vi "Drive_Hardware_Begin.vi"() -> ()   [LabVIEW 2019]
uses:
  <vilib>/Rock Robotics/WPI/ThirdParty/Phoenix-LabVIEW/Motor Controller/Controls/CTRE_Phoenix_MotorControl_BaseConfigurables.ctl
  <vilib>/Rock Robotics/WPI/ThirdParty/Phoenix-LabVIEW/Motor Controller/Controls/CTRE_Phoenix_MotorControl_VelocityMeasurementPeriod.ctl
  <vilib>/Rock Robotics/WPI/ThirdParty/Phoenix-LabVIEW/Motor Controller/Controls/CTRE_Phoenix_MotorControl_SlotStructure.ctl
  <vilib>/Rock Robotics/WPI/ThirdParty/Phoenix-LabVIEW/Motor Controller/Controls/CTRE_Phoenix_MotorControl_FilterStruct.ctl
  <vilib>/Rock Robotics/WPI/ThirdParty/Phoenix-LabVIEW/Motor Controller/Controls/CTRE_Phoenix_MotorControl_RemoteSourceType.ctl
  <vilib>/Rock Robotics/WPI/ThirdParty/Phoenix-LabVIEW/Controls/CTRE_Phoenix_CustomParamConfiguration.ctl
  <vilib>/Rock Robotics/WPI/ThirdParty/Phoenix-LabVIEW/Motor Controller/Controls/CTRE_Phoenix_MotorControl_FeedbackDevice_TalonFX.ctl
  <vilib>/Rock Robotics/WPI/ThirdParty/Phoenix-LabVIEW/Motor Controller/Controls/CTRE_Phoenix_MotorControl_LimitSwitchNormal.ctl
  <vilib>/Rock Robotics/WPI/ThirdParty/Phoenix-LabVIEW/Motor Controller/Controls/CTRE_Phoenix_MotorControl_LimitSwitchSource_Local.ctl
  <vilib>/Rock Robotics/WPI/ThirdParty/Phoenix-LabVIEW/Motor Controller/Controls/CTRE_Phoenix_MotorControl_SupplyCurrentLimitConfiguration.ctl
  <vilib>/Rock Robotics/WPI/ThirdParty/Phoenix-LabVIEW/Motor Controller/Controls/CTRE_Phoenix_MotorControl_StatorCurrentLimitConfiguration.ctl
  <vilib>/Rock Robotics/WPI/ThirdParty/Phoenix-LabVIEW/Motor Controller/Controls/CTRE_Phoenix_MotorControl_MotorCommutation_TalonFX.ctl
  <vilib>/Rock Robotics/WPI/ThirdParty/Phoenix-LabVIEW/CANCoder/Controls/CTRE_Phoenix_CANcoder_AbsoluteSensorRange.ctl
  <vilib>/Rock Robotics/WPI/ThirdParty/Phoenix-LabVIEW/CANCoder/Controls/CTRE_Phoenix_CANcoder_SensorInitializationStrategy.ctl
  <vilib>/Rock Robotics/WPI/ThirdParty/Phoenix-LabVIEW/Motor Controller/Controls/CTRE_Phoenix_MotorControl_TalonFXInvertType.ctl
  <vilib>/Rock Robotics/WPI/ThirdParty/Phoenix-LabVIEW/Motor Controller/Controls/CTRE_Phoenix_MotorControl_NeutralMode.ctl
  <vilib>/Rock Robotics/WPI/ThirdParty/Phoenix-LabVIEW/Pigeon IMU/CTRE_PigeonIMU_Open_TalonSRX.vi
  Globals/Drive_Globals.vi
panel:
  in  "Talon FX Configurables":T15={"Base Configurables"={"openLoopRamp"=0.0, "closedLoopRamp"=0.0, "peakOutputForward"=1.0, "peakOutputReverse"=-1.0, "nominalOutputForward"=0.0, "nominalOutputReverse"=0.0, "neutralDeadband"=0.0, "voltageCompSaturation"=0.0, "voltageMeasurementFilter"=32, "velocityMeasurementPeriod"=100, "velocityMeasurementWindow"=64, "forwardSoftLimitThreshold"=0, "reverseSoftLimitThreshold"=0, "forwardSoftLimitEnable"=FALSE, "reverseSoftLimitEnable"=FALSE, "slot0"={"P"=0.0, "I"=0.0, "D"=0.0, "F"=0.0, "integralZone"=0.0, "allowableClosedLoopError"=0, "maxIntegralAccumulator"=0.0, "closedLoopPeakOutput"=1.0, "closedLoopPeriod"=1}, "slot1"={"P"=0.0, "I"=0.0, "D"=0.0, "F"=0.0, "integralZone"=0.0, "allowableClosedLoopError"=0, "maxIntegralAccumulator"=0.0, "closedLoopPeakOutput"=1.0, "closedLoopPeriod"=1}, "slot2"={"P"=0.0, "I"=0.0, "D"=0.0, "F"=0.0, "integralZone"=0.0, "allowableClosedLoopError"=0, "maxIntegralAccumulator"=0.0, "closedLoopPeakOutput"=1.0, "closedLoopPeriod"=1}, "slot3"={"P"=0.0, "I"=0.0, "D"=0.0, "F"=0.0, "integralZone"=0.0, "allowableClosedLoopError"=0, "maxIntegralAccumulator"=0.0, "closedLoopPeakOutput"=1.0, "closedLoopPeriod"=1}, "auxPIDPolarity"=FALSE, "remoteFilter0"={"remoteSensorDeviceID"=0, "remoteSensorSource"=enum."Off"}, "remoteFilter1"={"remoteSensorDeviceID"=0, "remoteSensorSource"=enum."Off"}, "motionCruiseVelocity"=0, "motionAcceleration"=0, "motionProfileTrajectoryPeriod"=0, "feedbackNotContinuous"=FALSE, "remoteSensorClosedLoopDisableNeutralOnLOS"=FALSE, "clearPositionOnLimitF"=FALSE, "clearPositionOnLimitR"=FALSE, "clearPositionOnQuadIdx"=FALSE, "limitSwitchDisableNeutralOnLOS"=FALSE, "softLimitDisableNeutralOnLOS"=FALSE, "pulseWidthPeriod_EdgesPerRot"=1, "pulseWidthPeriod_FilterWindowSz"=1, "customParam"={"customParam0"=0, "customParam1"=0}, "trajectoryInterpolationEnable"=TRUE}, "primaryPID"={"selectedFeedbackCoefficient"=1.0, "selectedFeedbackSensor"=1}, "auxiliaryPID"={"selectedFeedbackCoefficient"=1.0, "selectedFeedbackSensor"=1}, "forwardLimitSwitchNormal"=enum."Normally Open", "reverseLimitSwitchNormal"=enum."Normally Open", "forwardLimitSwitchDeviceID"=0, "reverseLimitSwitchDeviceID"=0, "forwardLimitSwitchSource"=enum."Feedback Connector", "reverseLimitSwitchSource"=enum."Feedback Connector", "sum0Term"=1, "sum1Term"=1, "diff0Term"=1, "diff1Term"=1, "Supply Current Limit Configuration"={"Enable?"=FALSE, "Current Limit"=0.0, "Threshold Current"=0.0, "Threshold Time"=0.0}, "Stator Current Limit Configuration"={"Enable?"=FALSE, "Current Limit"=0.0, "Threshold Current"=0.0, "Threshold Time"=0.0}, "Motor Commutation"=enum."Trapezoidal", "Absolute Sensor Range"=enum."Unsigned [0 to 360)", "Integrated Sensor Offset (Degrees)"=0.0, "Sensor Initialization Strategy"=enum."Boot To Zero"} {"Base Configurables"."velocityMeasurementPeriod" items=["Period_1ms"=1, "Period_2ms"=2, "Period_5ms"=5, "Period_10ms"=10, "Period_20ms"=20, "Period_25ms"=25, "Period_50ms"=50, "Period_100ms"=100]; "primaryPID"."selectedFeedbackSensor" items=["Integrated Sensor"=1, "Sensor Sum (S0 + S1)"=9, "Sensor Difference (D0 - D1)"=10, "Remote Source 0"=11, "Remote Source 1"=12, "None"=14, "Software Emulated"=15]; "auxiliaryPID"."selectedFeedbackSensor" items=["Integrated Sensor"=1, "Sensor Sum (S0 + S1)"=9, "Sensor Difference (D0 - D1)"=10, "Remote Source 0"=11, "Remote Source 1"=12, "None"=14, "Software Emulated"=15]; "sum0Term" items=["Integrated Sensor"=1, "Sensor Sum (S0 + S1)"=9, "Sensor Difference (D0 - D1)"=10, "Remote Source 0"=11, "Remote Source 1"=12, "None"=14, "Software Emulated"=15]; "sum1Term" items=["Integrated Sensor"=1, "Sensor Sum (S0 + S1)"=9, "Sensor Difference (D0 - D1)"=10, "Remote Source 0"=11, "Remote Source 1"=12, "None"=14, "Software Emulated"=15]; "diff0Term" items=["Integrated Sensor"=1, "Sensor Sum (S0 + S1)"=9, "Sensor Difference (D0 - D1)"=10, "Remote Source 0"=11, "Remote Source 1"=12, "None"=14, "Software Emulated"=15]; "diff1Term" items=["Integrated Sensor"=1, "Sensor Sum (S0 + S1)"=9, "Sensor Difference (D0 - D1)"=10, "Remote Source 0"=11, "Remote Source 1"=12, "None"=14, "Software Emulated"=15]}
  # "False: Primary Output = PID[0] + PID[1]  ---  Auxiliary Output = PID[0] - PID[1]\nTrue:  Primary Output = PID[0] - PID[1] --- Auxiliary Output = PID[0] + PID[1]"
  # "Enable the motion profile executor to perform linear interpolation between profile points.  Defaults to True."
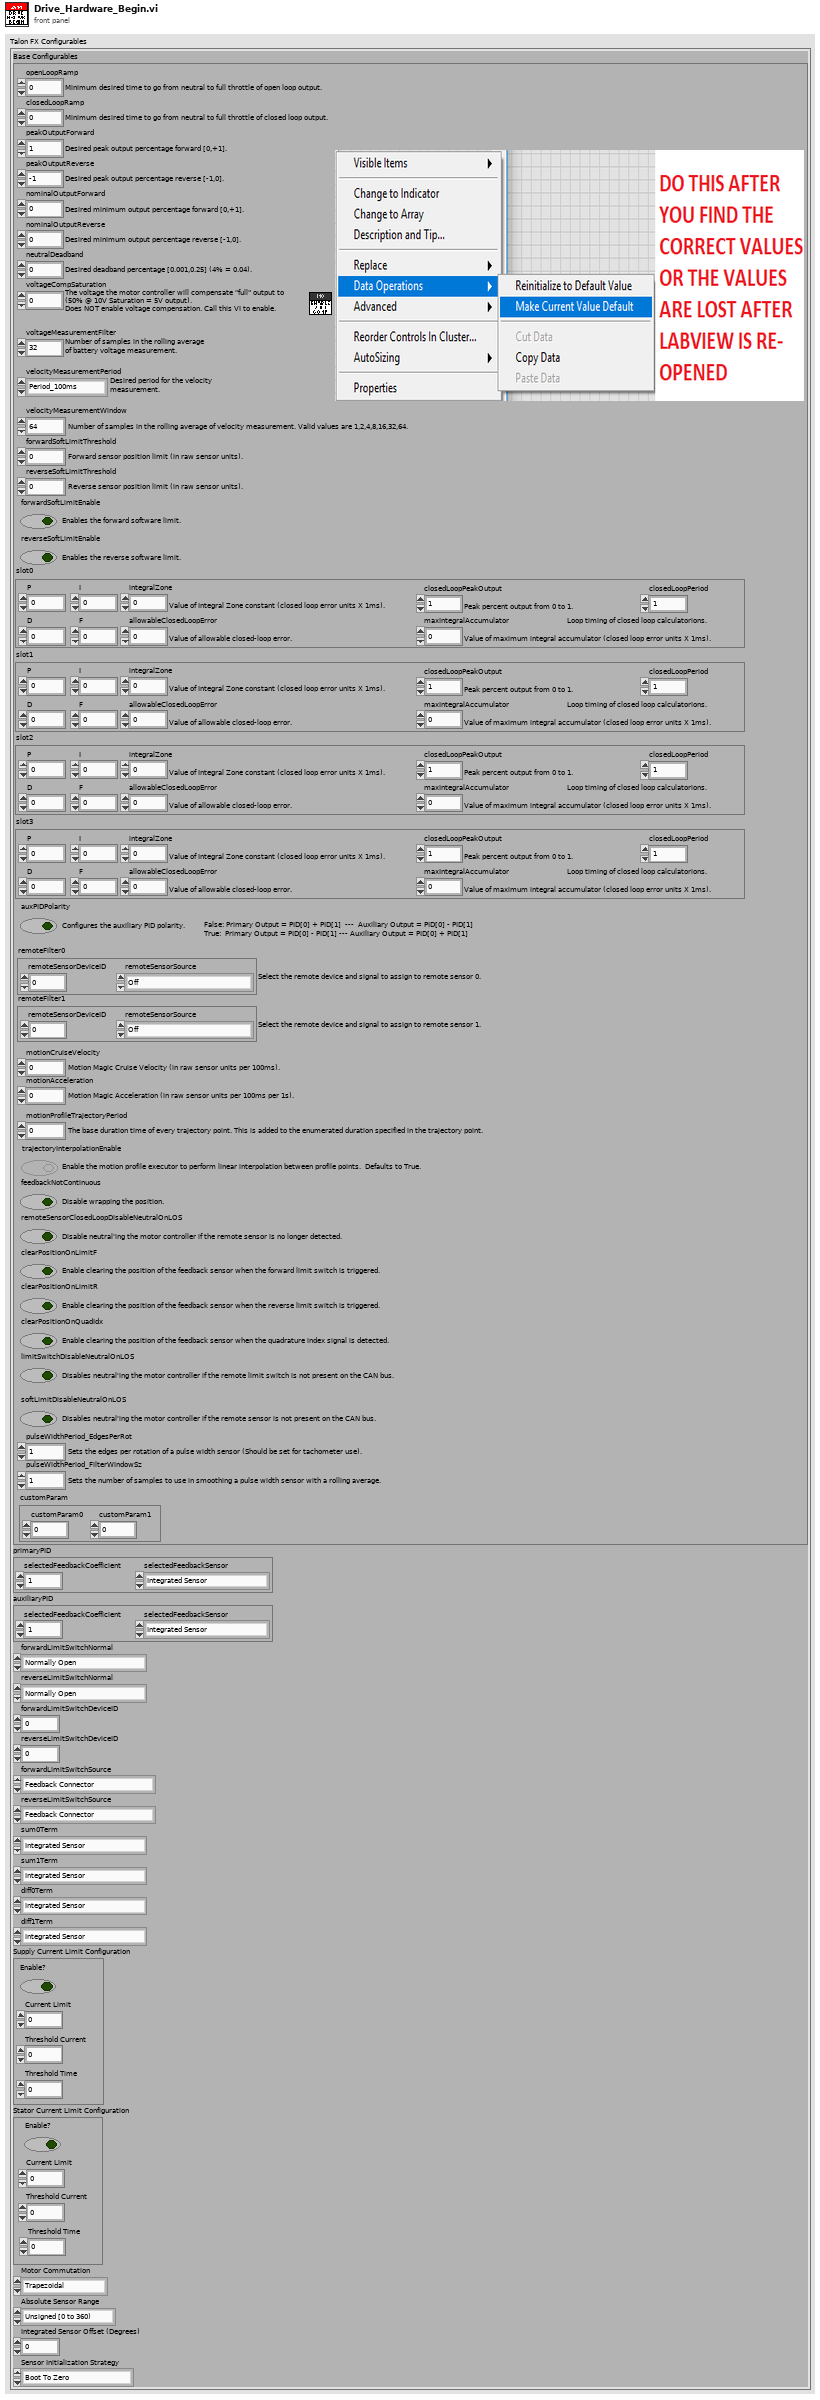
[diagram p1: front panel]
types:
  T1 = typedef "CTRE_Phoenix_MotorControl_BaseConfigurables.ctl" = cluster{"openLoopRamp":dbl, "closedLoopRamp":dbl, "peakOutputForward":dbl, "peakOutputReverse":dbl, "nominalOutputForward":dbl, "nominalOutputReverse":dbl, "neutralDeadband":dbl, "voltageCompSaturation":dbl, "voltageMeasurementFilter":i32, "velocityMeasurementPeriod":T2, "velocityMeasurementWindow":i32, "forwardSoftLimitThreshold":i32, "reverseSoftLimitThreshold":i32, "forwardSoftLimitEnable":bool, "reverseSoftLimitEnable":bool, "slot0":T3, "slot1":T3, "slot2":T3, "slot3":T3, "auxPIDPolarity":bool, "remoteFilter0":T4, "remoteFilter1":T4, "motionCruiseVelocity":i32, "motionAcceleration":i32, "motionProfileTrajectoryPeriod":i32, "feedbackNotContinuous":bool, "remoteSensorClosedLoopDisableNeutralOnLOS":bool, "clearPositionOnLimitF":bool, "clearPositionOnLimitR":bool, "clearPositionOnQuadIdx":bool, "limitSwitchDisableNeutralOnLOS":bool, "softLimitDisableNeutralOnLOS":bool, "pulseWidthPeriod_EdgesPerRot":i32, "pulseWidthPeriod_FilterWindowSz":i32, "customParam":T6, "trajectoryInterpolationEnable":bool}
  T2 = typedef "CTRE_Phoenix_MotorControl_VelocityMeasurementPeriod.ctl" = u16
  T3 = typedef "CTRE_Phoenix_MotorControl_SlotStructure.ctl" = cluster{"P":dbl, "I":dbl, "D":dbl, "F":dbl, "integralZone":dbl, "allowableClosedLoopError":i32, "maxIntegralAccumulator":dbl, "closedLoopPeakOutput":dbl, "closedLoopPeriod":i32}
  T4 = typedef "CTRE_Phoenix_MotorControl_FilterStruct.ctl" = cluster{"remoteSensorDeviceID":u8, "remoteSensorSource":T5}
  T5 = typedef "CTRE_Phoenix_MotorControl_RemoteSourceType.ctl" = enum16{"Off", "Talon SRX Selected Sensor", "Pigeon IMU Yaw", "Pigeon IMU Pitch", "Pigeon IMU Roll", "CANifier Quadrature", "CANifier PWM Input 0", "CANifier PWM Input 1", "CANifier PWM Input 2", "CANifier PWM Input 3", "Gadgeteer Pigeon Yaw", "Gadgeteer Pigeon Pitch", "Gadgeteer Pigeon Roll", "CANCoder"}
  T6 = typedef "CTRE_Phoenix_CustomParamConfiguration.ctl" = cluster{"customParam0":i32, "customParam1":i32}
  T7 = typedef "CTRE_Phoenix_MotorControl_FeedbackDevice_TalonFX.ctl" = i8
  T8 = typedef "CTRE_Phoenix_MotorControl_LimitSwitchNormal.ctl" = enum16{"Normally Open", "Normally Closed", "Disabled"}
  T9 = typedef "CTRE_Phoenix_MotorControl_LimitSwitchSource_Local.ctl" = enum16{"Feedback Connector", "Remote Talon SRX", "Remote CANifier", "Deactivated"}
  T10 = typedef "CTRE_Phoenix_MotorControl_SupplyCurrentLimitConfiguration.ctl" = cluster{"Enable?":bool, "Current Limit":dbl, "Threshold Current":dbl, "Threshold Time":dbl}
  T11 = typedef "CTRE_Phoenix_MotorControl_StatorCurrentLimitConfiguration.ctl" = cluster{"Enable?":bool, "Current Limit":dbl, "Threshold Current":dbl, "Threshold Time":dbl}
  T12 = typedef "CTRE_Phoenix_MotorControl_MotorCommutation_TalonFX.ctl" = enum16{"Trapezoidal"}
  T13 = typedef "CTRE_Phoenix_CANcoder_AbsoluteSensorRange.ctl" = enum16{"Unsigned [0 to 360)", "Signed [-180 to +180)"}
  T14 = typedef "CTRE_Phoenix_CANcoder_SensorInitializationStrategy.ctl" = enum16{"Boot To Zero", "Boot To Absolute Position"}
  T15 = cluster{"Base Configurables":T1, "primaryPID":cluster{"selectedFeedbackCoefficient":dbl, "selectedFeedbackSensor":T7}, "auxiliaryPID":cluster{"selectedFeedbackCoefficient":dbl, "selectedFeedbackSensor":T7}, "forwardLimitSwitchNormal":T8, "reverseLimitSwitchNormal":T8, "forwardLimitSwitchDeviceID":i32, "reverseLimitSwitchDeviceID":i32, "forwardLimitSwitchSource":T9, "reverseLimitSwitchSource":T9, "sum0Term":T7, "sum1Term":T7, "diff0Term":T7, "diff1Term":T7, "Supply Current Limit Configuration":T10, "Stator Current Limit Configuration":T11, "Motor Commutation":T12, "Absolute Sensor Range":T13, "Integrated Sensor Offset (Degrees)":dbl, "Sensor Initialization Strategy":T14}
  T16 = typedef "CTRE_Phoenix_MotorControl_TalonFXInvertType.ctl" = enum16{"Counter-Clockwise", "Clockwise"}
  T17 = typedef "CTRE_Phoenix_MotorControl_NeutralMode.ctl" = enum8{"EEPROMSetting", "Override to Coast", "Override to Brake"}
  T18 = typedef "WPI_MotorControlDeviceRef.ctl" = cluster{"DeviceStatus":errorcluster, "Type":T19, "PWM":cluster{"PWM Channel":T20, "DeadBand":T21}, "CAN":cluster{"Device Number":u8, "SetOutput VI Ref":variant, "GetOutput VI Ref":variant, "Enable VI Ref":variant, "Disable VI Ref":variant, "Data":variant}, "Invert":bool, "DIO PWM":cluster{"PWM \"Enable\" Channel":T20, "DIOChannel":T22, "PWM Rate":dbl}}
  T19 = typedef "WPI_MotorControlType.ctl" = enum16{"PWM", "CAN", "DIO PWM"}
  T20 = typedef "FPGA_DIOPWMChannel.ctl" = enum8{"PWM 0", "PWM 1", "PWM 2", "PWM 3", "PWM 4", "PWM 5", "PWM 6", "PWM 7", "PWM 8", "PWM 9", "PWM MXP 0", "PWM MXP 1", "PWM MXP 2", "PWM MXP 3", "PWM MXP 4", "PWM MXP 5", "PWM MXP 6", "PWM MXP 7", "PWM MXP 8", "PWM MXP 9", "Invalid"}
  T21 = typedef "WPI_PWMDeadband.ctl" = cluster{"Name":string, "maxPositivePwm":i32, "minPositivePwm":i32, "centerPwm":i32, "maxNegativePwm":i32, "minNegativePwm":i32, "angularRange":u16}
  T22 = typedef "FPGA_DIOChannel.ctl" = enum8{"DIO 0", "DIO 1", "DIO 2", "DIO 3", "DIO 4", "DIO 5", "DIO 6", "DIO 7", "DIO 8", "DIO 9", "DIO MXP 0", "DIO MXP 1", "DIO MXP 2", "DIO MXP 3", "DIO MXP 4", "DIO MXP 5", "DIO MXP 6", "DIO MXP 7", "DIO MXP 8", "DIO MXP 9", "DIO MXP 10", "DIO MXP 11", "DIO MXP 12", "DIO MXP 13", "DIO MXP 14", "DIO MXP 15", "SPI Port CS1", "SPI Port CS2", "SPI Port CS3", "SPI Port MISO", "SPI Port MOSI", "Invalid"}
  T23 = typedef "CTRE_PigeonIMU_DeviceRef.ctl" = cluster{"DeviceStatus":errorcluster, "Device Number":u8, "Type":T24, "Device ID":u32, "Handle":u64, "UsageFrame":u32, "Library Path":path}
  T24 = typedef "CTRE_PigeonIMU_ConnectionType.ctl" = u32
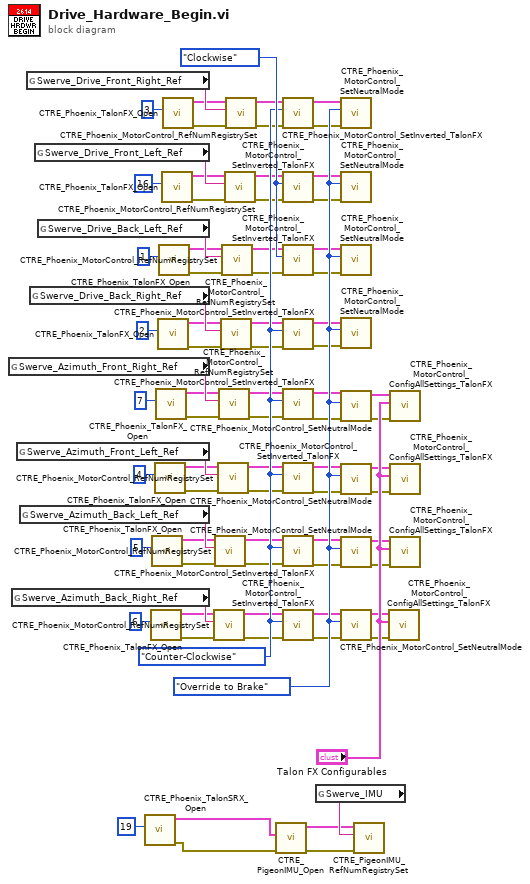
[diagram p0: block diagram]
diagram:
  w82 = CTRE_Phoenix_MotorControl_TalonFXInvertType."Clockwise" ("Invert Type")
  w69 = CTRE_Phoenix_MotorControl_NeutralMode."Override to Brake" ("Motor Control Neutral Mode")
  w51 = CTRE_Phoenix_MotorControl_TalonFXInvertType."Counter-Clockwise" ("Invert Type")
  n1 = global read "Drive_Globals.vi" "Swerve_Azimuth_Front_Right_Ref"() -> (w47:string)
  n2 = global read "Drive_Globals.vi" "Swerve_Azimuth_Back_Right_Ref"() -> (w50:string)
  n3 = global read "Drive_Globals.vi" "Swerve_Azimuth_Front_Left_Ref"() -> (w48:string)
  n4 = global read "Drive_Globals.vi" "Swerve_Azimuth_Back_Left_Ref"() -> (w49:string)
  n5 = global read "Drive_Globals.vi" "Swerve_Drive_Front_Right_Ref"() -> (w43:string)
  n6 = global read "Drive_Globals.vi" "Swerve_Drive_Back_Right_Ref"() -> (w46:string)
  n7 = global read "Drive_Globals.vi" "Swerve_Drive_Front_Left_Ref"() -> (w44:string)
  n8 = global read "Drive_Globals.vi" "Swerve_Drive_Back_Left_Ref"() -> (w45:string)
  n9 = call <vilib>:"CTRE_Phoenix_TalonSRX_Open.vi"("Device Number"=u8 19) -> ("error out"=w72:errorcluster, "CAN Talon SRX Ref"=w71:T18)  [unwired: 9 in]
  n10 = call <vilib>:"CTRE_Phoenix_TalonFX_Open.vi"("Device Number"=u8 6) -> ("error out"=w29:errorcluster, "CAN Talon SRX Ref"=w32:T18)  [unwired: 9 in]
  n11 = call <vilib>:"CTRE_Phoenix_TalonFX_Open.vi"("Device Number"=u8 5) -> ("error out"=w26:errorcluster, "CAN Talon SRX Ref"=w23:T18)  [unwired: 9 in]
  n12 = call <vilib>:"CTRE_Phoenix_TalonFX_Open.vi"("Device Number"=u8 4) -> ("error out"=w36:errorcluster, "CAN Talon SRX Ref"=w33:T18)  [unwired: 9 in]
  n13 = call <vilib>:"CTRE_Phoenix_TalonFX_Open.vi"("Device Number"=u8 7) -> ("error out"=w39:errorcluster, "CAN Talon SRX Ref"=w42:T18)  [unwired: 9 in]
  n14 = call <vilib>:"CTRE_Phoenix_TalonFX_Open.vi"("Device Number"=u8 2) -> ("error out"=w16:errorcluster, "CAN Talon SRX Ref"=w13:T18)  [unwired: 9 in]
  n15 = call <vilib>:"CTRE_Phoenix_TalonFX_Open.vi"("Device Number"=u8 1) -> ("error out"=w19:errorcluster, "CAN Talon SRX Ref"=w22:T18)  [unwired: 9 in]
  n16 = call <vilib>:"CTRE_Phoenix_TalonFX_Open.vi"("Device Number"=u8 16) -> ("error out"=w9:errorcluster, "CAN Talon SRX Ref"=w12:T18)  [unwired: 9 in]
  n17 = call <vilib>:"CTRE_Phoenix_TalonFX_Open.vi"("Device Number"=u8 3) -> ("error out"=w6:errorcluster, "CAN Talon SRX Ref"=w3:T18)  [unwired: 9 in]
  n18 = call <vilib>:"CTRE_Phoenix_MotorControl_RefNumRegistrySet.vi"("error in (no error)"=w29, "refnum name"=w50, "PhoenixMotorControlDevRef"=w32) -> ("error out"=w30:errorcluster, "PhoenixMotorControlDevRef"=w31:T18)  [unwired: 7 in]
  n19 = call <vilib>:"CTRE_Phoenix_MotorControl_RefNumRegistrySet.vi"("error in (no error)"=w26, "refnum name"=w49, "PhoenixMotorControlDevRef"=w23) -> ("error out"=w25:errorcluster, "PhoenixMotorControlDevRef"=w24:T18)  [unwired: 7 in]
  n20 = call <vilib>:"CTRE_Phoenix_MotorControl_RefNumRegistrySet.vi"("error in (no error)"=w36, "refnum name"=w48, "PhoenixMotorControlDevRef"=w33) -> ("error out"=w35:errorcluster, "PhoenixMotorControlDevRef"=w34:T18)  [unwired: 7 in]
  n21 = call <vilib>:"CTRE_Phoenix_MotorControl_RefNumRegistrySet.vi"("error in (no error)"=w39, "refnum name"=w47, "PhoenixMotorControlDevRef"=w42) -> ("error out"=w40:errorcluster, "PhoenixMotorControlDevRef"=w41:T18)  [unwired: 7 in]
  n22 = call <vilib>:"CTRE_Phoenix_MotorControl_RefNumRegistrySet.vi"("error in (no error)"=w16, "refnum name"=w46, "PhoenixMotorControlDevRef"=w13) -> ("error out"=w15:errorcluster, "PhoenixMotorControlDevRef"=w14:T18)  [unwired: 7 in]
  n23 = call <vilib>:"CTRE_Phoenix_MotorControl_RefNumRegistrySet.vi"("error in (no error)"=w19, "refnum name"=w45, "PhoenixMotorControlDevRef"=w22) -> ("error out"=w20:errorcluster, "PhoenixMotorControlDevRef"=w21:T18)  [unwired: 7 in]
  n24 = call <vilib>:"CTRE_Phoenix_MotorControl_RefNumRegistrySet.vi"("error in (no error)"=w9, "refnum name"=w44, "PhoenixMotorControlDevRef"=w12) -> ("error out"=w10:errorcluster, "PhoenixMotorControlDevRef"=w11:T18)  [unwired: 7 in]
  n25 = call <vilib>:"CTRE_Phoenix_MotorControl_RefNumRegistrySet.vi"("error in (no error)"=w6, "refnum name"=w43, "PhoenixMotorControlDevRef"=w3) -> ("error out"=w5:errorcluster, "PhoenixMotorControlDevRef"=w4:T18)  [unwired: 7 in]
  n26 = call-poly <vilib>:"CTRE_PigeonIMU_Open.vi"("error in"=w72, "CAN Talon SRX Ref"=w71) -> ("error out"=w2:errorcluster, "PigeonIMUDevRef"=w1:T23)  [unwired: 8 in]
  n27 = call <vilib>:"CTRE_Phoenix_MotorControl_SetInverted_TalonFX.vi"("error in (no error)"=w5, "Invert Type"=w51, "PhoenixMotorControlDevRef"=w4) -> ("error out"=w56:errorcluster, "PhoenixMotorControlDevRef"=w55:T18)  [unwired: 7 in]
  n28 = call <vilib>:"CTRE_Phoenix_MotorControl_SetInverted_TalonFX.vi"("error in (no error)"=w10, "Invert Type"=w82, "PhoenixMotorControlDevRef"=w11) -> ("error out"=w58:errorcluster, "PhoenixMotorControlDevRef"=w57:T18)  [unwired: 7 in]
  n29 = call <vilib>:"CTRE_Phoenix_MotorControl_SetInverted_TalonFX.vi"("error in (no error)"=w20, "Invert Type"=w82, "PhoenixMotorControlDevRef"=w21) -> ("error out"=w60:errorcluster, "PhoenixMotorControlDevRef"=w59:T18)  [unwired: 7 in]
  n30 = call <vilib>:"CTRE_Phoenix_MotorControl_SetInverted_TalonFX.vi"("error in (no error)"=w15, "Invert Type"=w51, "PhoenixMotorControlDevRef"=w14) -> ("error out"=w62:errorcluster, "PhoenixMotorControlDevRef"=w61:T18)  [unwired: 7 in]
  n31 = call <vilib>:"CTRE_Phoenix_MotorControl_SetInverted_TalonFX.vi"("error in (no error)"=w40, "Invert Type"=w51, "PhoenixMotorControlDevRef"=w41) -> ("error out"=w64:errorcluster, "PhoenixMotorControlDevRef"=w63:T18)  [unwired: 7 in]
  n32 = call <vilib>:"CTRE_Phoenix_MotorControl_SetInverted_TalonFX.vi"("error in (no error)"=w35, "Invert Type"=w51, "PhoenixMotorControlDevRef"=w34) -> ("error out"=w66:errorcluster, "PhoenixMotorControlDevRef"=w65:T18)  [unwired: 7 in]
  n33 = call <vilib>:"CTRE_Phoenix_MotorControl_SetInverted_TalonFX.vi"("error in (no error)"=w25, "Invert Type"=w51, "PhoenixMotorControlDevRef"=w24) -> ("error out"=w68:errorcluster, "PhoenixMotorControlDevRef"=w67:T18)  [unwired: 7 in]
  n34 = call <vilib>:"CTRE_Phoenix_MotorControl_SetInverted_TalonFX.vi"("error in (no error)"=w30, "Invert Type"=w51, "PhoenixMotorControlDevRef"=w31) -> ("error out"=w54:errorcluster, "PhoenixMotorControlDevRef"=w53:T18)  [unwired: 7 in]
  n35 = global read "Drive_Globals.vi" "Swerve_IMU"() -> (w52:string)
  n36 = call <vilib>:"CTRE_Phoenix_MotorControl_SetNeutralMode.vi"("error in (no error)"=w56, "Motor Control Neutral Mode"=w69, "PhoenixMotorControlDevRef"=w55) -> ()  [unwired: 7 in, 2 out]
  n37 = call <vilib>:"CTRE_Phoenix_MotorControl_SetNeutralMode.vi"("error in (no error)"=w58, "Motor Control Neutral Mode"=w69, "PhoenixMotorControlDevRef"=w57) -> ()  [unwired: 7 in, 2 out]
  n38 = call <vilib>:"CTRE_Phoenix_MotorControl_SetNeutralMode.vi"("error in (no error)"=w60, "Motor Control Neutral Mode"=w69, "PhoenixMotorControlDevRef"=w59) -> ()  [unwired: 7 in, 2 out]
  n39 = call <vilib>:"CTRE_Phoenix_MotorControl_SetNeutralMode.vi"("error in (no error)"=w62, "Motor Control Neutral Mode"=w69, "PhoenixMotorControlDevRef"=w61) -> ()  [unwired: 7 in, 2 out]
  n40 = call <vilib>:"CTRE_Phoenix_MotorControl_SetNeutralMode.vi"("error in (no error)"=w64, "Motor Control Neutral Mode"=w69, "PhoenixMotorControlDevRef"=w63) -> ("error out"=w79:errorcluster, "PhoenixMotorControlDevRef"=w80:T18)  [unwired: 7 in]
  n41 = call <vilib>:"CTRE_Phoenix_MotorControl_SetNeutralMode.vi"("error in (no error)"=w66, "Motor Control Neutral Mode"=w69, "PhoenixMotorControlDevRef"=w65) -> ("error out"=w77:errorcluster, "PhoenixMotorControlDevRef"=w78:T18)  [unwired: 7 in]
  n42 = call <vilib>:"CTRE_Phoenix_MotorControl_SetNeutralMode.vi"("error in (no error)"=w68, "Motor Control Neutral Mode"=w69, "PhoenixMotorControlDevRef"=w67) -> ("error out"=w76:errorcluster, "PhoenixMotorControlDevRef"=w75:T18)  [unwired: 7 in]
  n43 = call <vilib>:"CTRE_Phoenix_MotorControl_SetNeutralMode.vi"("error in (no error)"=w54, "Motor Control Neutral Mode"=w69, "PhoenixMotorControlDevRef"=w53) -> ("error out"=w74:errorcluster, "PhoenixMotorControlDevRef"=w73:T18)  [unwired: 7 in]
  n44 = call <vilib>:"CTRE_PigeonIMU_RefNumRegistrySet.vi"("error in (no error)"=w2, "refnum name"=w52, "PigeonIMUDevRef"=w1) -> ()  [unwired: 7 in, 2 out]
  n45 = call <vilib>:"CTRE_Phoenix_MotorControl_ConfigAllSettings_TalonFX.vi"("error in (no error)"=w74, "Talon FX Configurables"="Talon FX Configurables", "PhoenixMotorControlDevRef"=w73) -> ()  [unwired: 7 in, 2 out]
  n46 = call <vilib>:"CTRE_Phoenix_MotorControl_ConfigAllSettings_TalonFX.vi"("error in (no error)"=w79, "Talon FX Configurables"="Talon FX Configurables", "PhoenixMotorControlDevRef"=w80) -> ()  [unwired: 7 in, 2 out]
  n47 = call <vilib>:"CTRE_Phoenix_MotorControl_ConfigAllSettings_TalonFX.vi"("error in (no error)"=w77, "Talon FX Configurables"="Talon FX Configurables", "PhoenixMotorControlDevRef"=w78) -> ()  [unwired: 7 in, 2 out]
  n48 = call <vilib>:"CTRE_Phoenix_MotorControl_ConfigAllSettings_TalonFX.vi"("error in (no error)"=w76, "Talon FX Configurables"="Talon FX Configurables", "PhoenixMotorControlDevRef"=w75) -> ()  [unwired: 7 in, 2 out]
